vi "stringToarray.vi"(1 "String":string) -> (0 "Array":string[](array[string]))   [LabVIEW 2012]
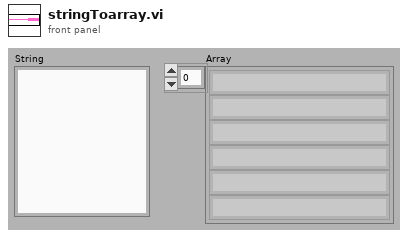
[diagram p1: front panel]
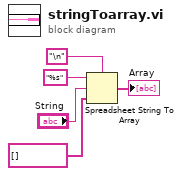
[diagram p0: block diagram]
diagram:
  n1 = Spreadsheet String To Array(delimiter (Tab)="\n", format string="%s" ("delimiter (Tab)"), spreadsheet string="String", array type (2D Dbl)=string[] []) -> (array=→"Array":string[])
